vi "cal8bit.vi"(9 "分辨率":string, 10 "Array":u8[](array[numeric])) -> (2 "ArrayOut":u8[](array[numeric]))   [LabVIEW 2016]
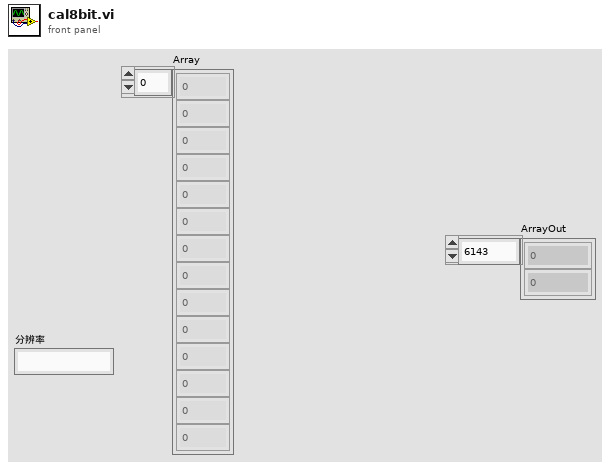
[diagram p1: front panel]
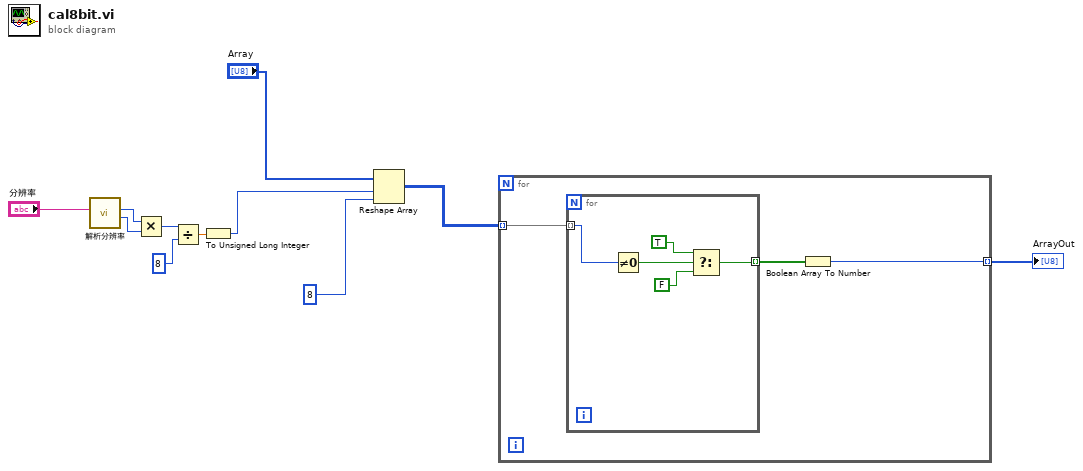
[diagram p0: block diagram]
diagram:
  n1 = call "解析分辨率.vi"("分辨率"="分辨率") -> ("number 2"=w5:i32, "number"=w6:i32)  [unwired: 9 in]
  n2 = Multiply(x=w6, y=w5) -> (x*y=w4:i32)
  n3 = Divide(x=w4, y=8) -> (x/y=w2:dbl)
  n4 = To Unsigned Long Integer(number=w2) -> (unsigned 32bit integer=w1:u32)
  n5 = Reshape Array("Array", w1, 8 ("dimension size")) -> (w9:u8[][])
  n6 = for {
    tunnel: w9 -> [w14] mode=indexing
    tunnel: [w12] -> w8 mode=indexing
    n7 = for {
      tunnel: w14 -> [w19] mode=indexing
      tunnel: [w15] -> w13 mode=indexing
      n8 = Not Equal To 0?(x=w19) -> (x != 0?=w17:bool)
      n9 = Select(t=TRUE, s=w17, f=FALSE) -> (s? t:f=w15:bool)
    }
    n10 = Boolean Array To Number(Boolean array=w13) -> (number=w12:u32)
  }
  "ArrayOut" <- w8
